vi "Vision Processor_modified.vi"(5 "error in":errorcluster, 7 "Image In":T2) -> (0 "error out":errorcluster, 3 "Image Out":T2(plugin-control))   [LabVIEW 2013]
uses:
  <vilib>/vision/Image Controls.llb/IMAQ Image.ctl
  <vilib>/vision/NI_Vision_Development_Module.lvlib
panel:
  out "HSL Histogram":T1(graph)
  out "Image In":T2(plugin-control)
  # "0  center of mass x\n1  center of mass y\n2  first pixel x\n3  first pixel y\n4  bounding rect left\n5  bounding rect top\n6  bounding rect right\n7  bounding rect bottom\n8 max feret diameter start x\n9  max feret diameter start y\n10 max feret diameter end x\n11 max feret diameter end y\n12 max horiz segment length left\n13 max horiz segment length right\n14 max horiz segment length row\n15 bounding rect width \n16 bounding rect height\n17 bounding rect diagional\n..\n33 area"
  # "13'3\"\n3'9\""
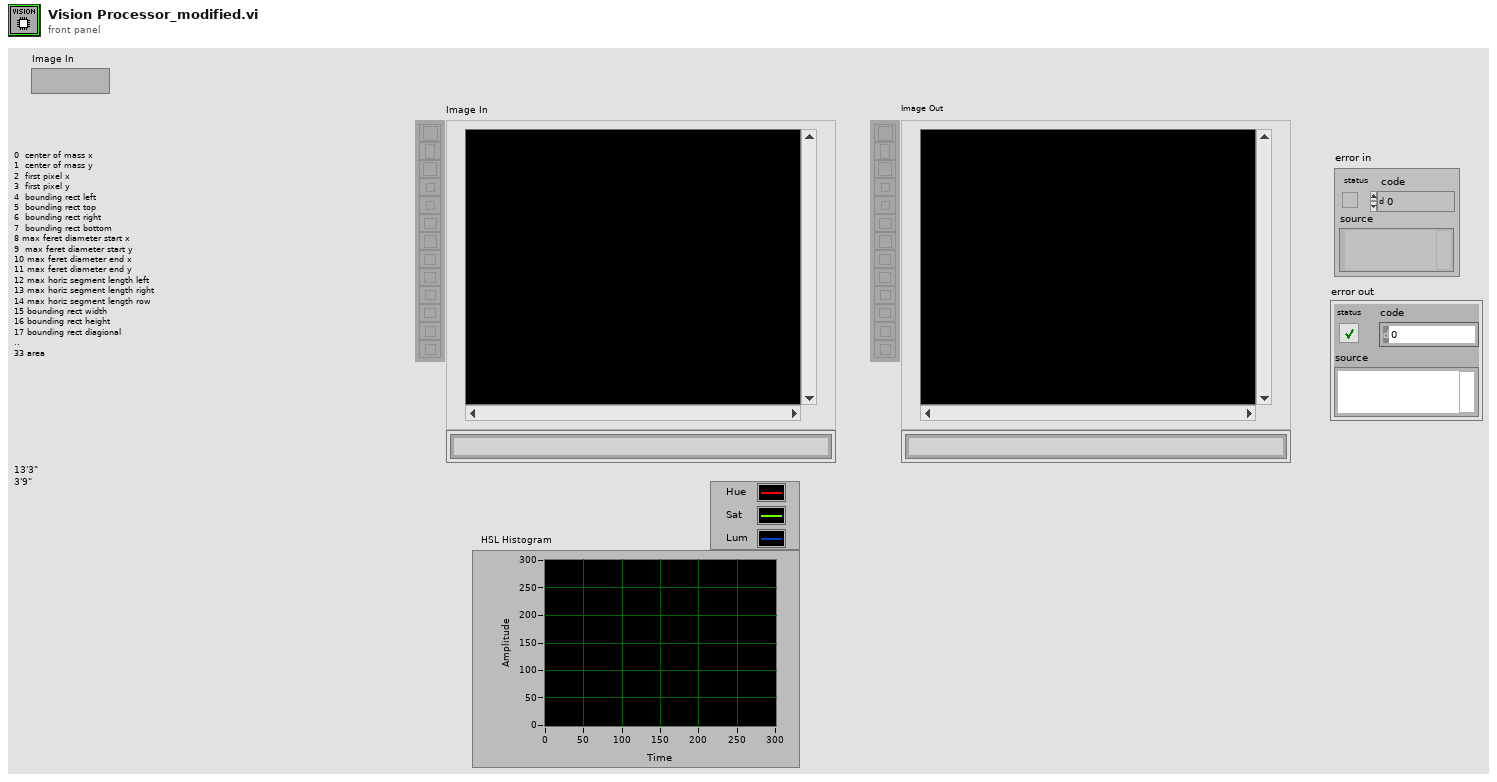
[diagram p1: front panel]
types:
  T1 = cluster{"Starting Value":sgl, "Incremental Value":sgl, "Histogram":u32[]}[]
  T2 = typedef "IMAQ Image.ctl" = refnum<image>
  T3 = enum32{"AutoM", "Close", "Dilate", "Erode", "Gradient", "Gradient out", "Gradient in", "Hit miss", "Open", "PClose", "POpen", "Thick", "Thin"}
  T4 = typedef "Image Type" = u32
  T5 = cluster{"Starting Value":sgl, "Incremental Value":sgl, "Histogram":u32[]}
  T6 = typedef "Particle Parameters" = i32
  T7 = cluster{"Measurement Parameter":T6, "Range Lower Value":dbl, "Range Upper Value":dbl, "Range":bool, "Measurement Type":bool}[]
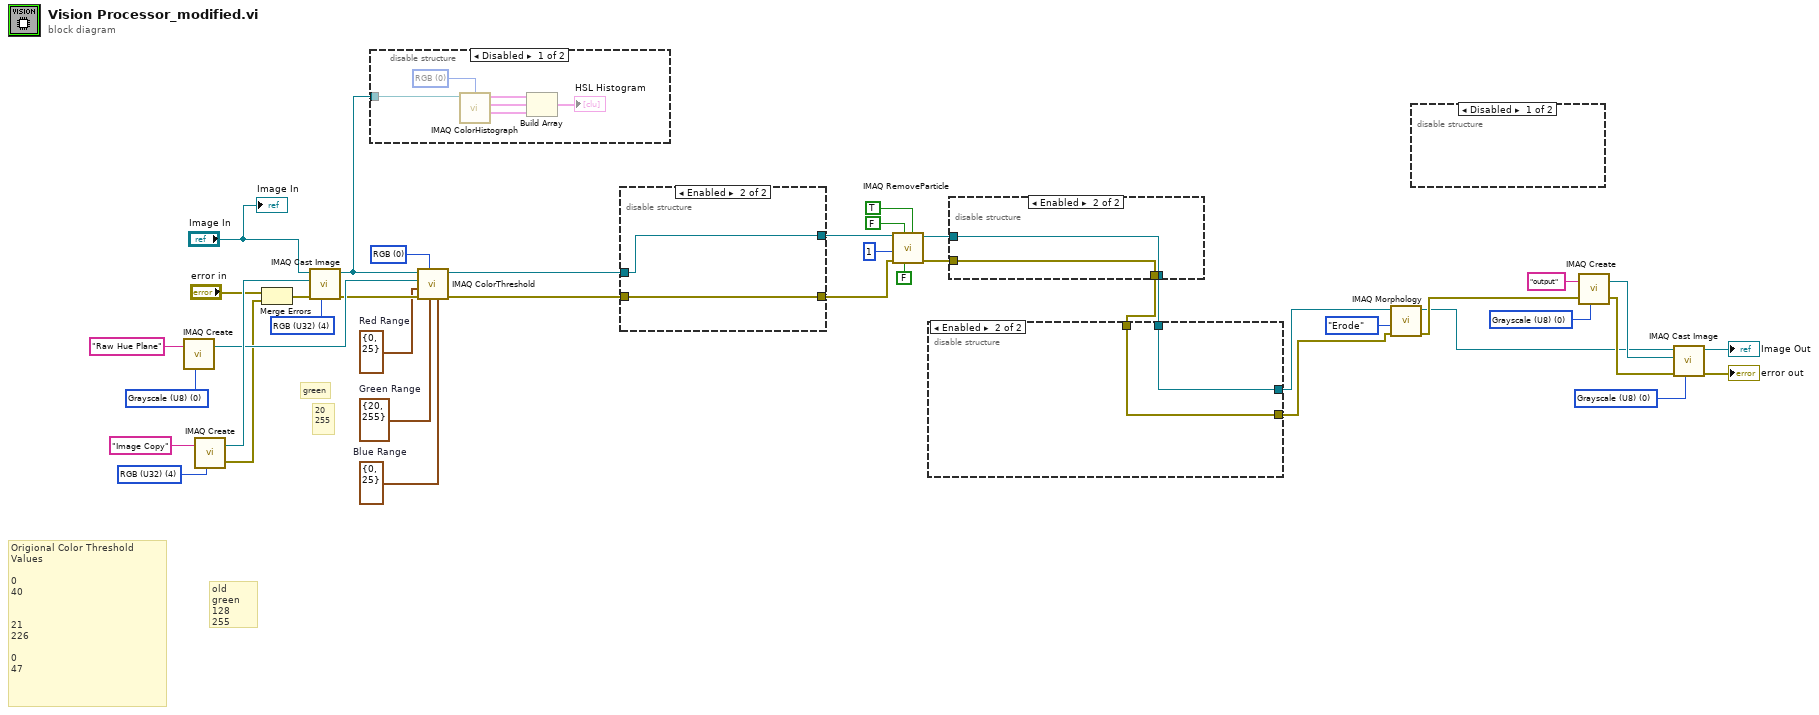
[diagram p0: block diagram]
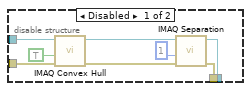
[diagram p2: hidden frame]
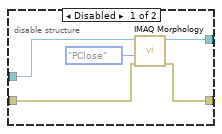
[diagram p3: hidden frame]
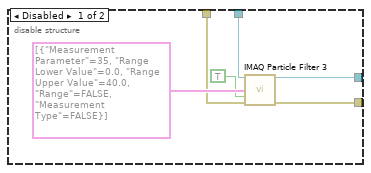
[diagram p5: hidden frame]
diagram:
  w12 = T4 0 items=["Grayscale (U8)", "Grayscale (I16)", "Grayscale (SGL)", "Complex (CSG)", "RGB (U32)", "HSL (U32)", "RGB (U64)", "Grayscale (U16)"] ("Image Type")
  w24 = T4 0 items=["Grayscale (U8)", "Grayscale (I16)", "Grayscale (SGL)", "Complex (CSG)", "RGB (U32)", "HSL (U32)", "RGB (U64)", "Grayscale (U16)"] ("Image Type")
  w25 = cluster{"Lower value":i32, "Upper value":i32} {"Lower value"=0, "Upper value"=25}  # Blue Range
  w28 = cluster{"Lower value":i32, "Upper value":i32} {"Lower value"=0, "Upper value"=25}  # Red Range
  w31 = cluster{"Lower value":i32, "Upper value":i32} {"Lower value"=20, "Upper value"=255}  # Green Range
  w29 = u16 0 items=["RGB", "HSL", "HSV", "HSI"] ("Color Mode")
  w37 = T4 0 items=["Grayscale (U8)", "Grayscale (I16)", "Grayscale (SGL)", "Complex (CSG)", "RGB (U32)", "HSL (U32)", "RGB (U64)", "Grayscale (U16)"] ("Image Type")
  w39 = T4 4 items=["Grayscale (U8)", "Grayscale (I16)", "Grayscale (SGL)", "Complex (CSG)", "RGB (U32)", "HSL (U32)", "RGB (U64)", "Grayscale (U16)"] ("Image Type")
  w40 = T4 4 items=["Grayscale (U8)", "Grayscale (I16)", "Grayscale (SGL)", "Complex (CSG)", "RGB (U32)", "HSL (U32)", "RGB (U64)", "Grayscale (U16)"] ("Image Type")
  # "old green\n128\n255"
  # "green"
  # "20\n255"
  # "Origional Color Threshold Values\n\n0\n40\n\n\n21\n226\n\n0\n47"
  n1 = call "IMAQ Create"("Image Name"="Raw Hue Plane", "Image Type"=w37) -> ("New Image"=w33:T2)  [unwired: 3 in, 1 out]
  n2 = call "IMAQ Create"("Image Name"="Image Copy", "Image Type"=w40) -> ("New Image"=w36:T2, "error out"=w26:errorcluster)  [unwired: 3 in]
  n3 = Merge Errors("error in", w26) -> (w27:errorcluster)
  n4 = call "IMAQ Cast Image"("Image Type"=w39, "error in (no error)"=w27, "Image Dst"=w36, "Image Src"="Image In") -> ("error out"=w30:errorcluster, "Image Dst Out"=w32:T2)  [unwired: 6 in]
  n5 = disable-structure shown="Disabled" {
    disable-tunnel: w32 -> [w42 _]
    frame Disabled {
      w43 = u16 0 items=["RGB", "HSL", "HSV", "HSI"] ("Color Mode")
      n6 = call "IMAQ ColorHistograph"("Color Mode"=w43, "Image Src"=w42) -> ("Red or Hue Histogram Graph"=w47:T5, "Green or Sat Histogram Graph"=w46:T5, "Blue or Luma or Val or Inten Histogram Graph"=w45:T5)  [unwired: 4 in, 1 out]
      n7 = Build Array(w47, w46, w45) -> (→"HSL Histogram":T1)
    }
    frame Enabled {
    }
  }
  n8 = call "IMAQ ColorThreshold"("Blue or Luma or Val or Inten Range"=w25, "Green or Sat Range"=w31, "Color Mode"=w29, "error in (no error)"=w30, "Red or Hue Range"=w28, "Image Dst"=w33, "Image Src"=w32) -> ("error out"=w16:errorcluster, "Image Dst Out"=w17:T2)  [unwired: 3 in]
  n9 = disable-structure shown="Enabled" {
    disable-tunnel: [w51 w54] -> w18
    disable-tunnel: w17 -> [w50 w54]
    disable-tunnel: w16 -> [w49 w53]
    disable-tunnel: [w48 w53] -> w15
    frame Disabled {
      n10 = call "IMAQ Morphology"("error in (no error)"=w49, "Operation"=T3."PClose", "Image Src"=w50) -> ("error out"=w48:errorcluster, "Image Dst Out"=w51:T2)  [unwired: 7 in]
    }
    frame Enabled {
    }
  }
  n11 = call "IMAQ RemoveParticle"("Connectivity 4/8 (8)"=TRUE, "Low Pass/High Pass (Low)"=FALSE, "Square/Hexa (Square)"=FALSE, "error in (no error)"=w15, "Number of Erosion"=1, "Image Src"=w18) -> ("error out"=w8:errorcluster, "Image Dst Out"=w9:T2)  [unwired: 1 in, 3 out]
  n12 = disable-structure shown="Enabled" {
    disable-tunnel: w9 -> [w61 w64]
    disable-tunnel: w8 -> [w60 w63]
    disable-tunnel: [w58 w64] -> w7
    disable-tunnel: [w55 w63] -> w6
    frame Disabled {
      n13 = call "IMAQ Convex Hull"("error in (no error)"=w60, "Connectivity 4/8 (8)"=TRUE, "Image Src"=w61) -> ("error out"=w56:errorcluster, "Image Dst Out"=w59:T2)  [unwired: 1 in, 6 out]
      n14 = call "IMAQ Separation"("error in (no error)"=w56, "Nb of Erosion"=1, "Image Src"=w59) -> ("error out"=w55:errorcluster, "Image Dst Out"=w58:T2)  [unwired: 7 in]
    }
    frame Enabled {
    }
  }
  n15 = disable-structure shown="Enabled" {
    disable-tunnel: w7 -> [w69 w72]
    disable-tunnel: [w67 w72] -> w3
    disable-tunnel: w6 -> [w66 w71]
    disable-tunnel: [w65 w71] -> w4
    frame Disabled {
      n16 = call "IMAQ Particle Filter 3"("Image Src"=w69, "Selection Values"=T7 [{"Measurement Parameter"=35, "Range Lower Value"=0.0, "Range Upper Value"=40.0, "Range"=FALSE, "Measurement Type"=FALSE}], "Keep/Remove Particles (F)"=TRUE, "error in (no error)"=w66) -> ("Image Dst Out"=w67:T2, "error out"=w65:errorcluster)  [unwired: 9 in, 1 out]
    }
    frame Enabled {
    }
  }
  n17 = call "IMAQ Morphology"("error in (no error)"=w4, "Operation"=T3."Erode", "Image Src"=w3) -> ("error out"=w2:errorcluster, "Image Dst Out"=w1:T2)  [unwired: 7 in]
  n18 = disable-structure shown="Disabled" {
    frame Disabled {
    }
    frame Enabled {
    }
  }
  n19 = call "IMAQ Create"("Image Name"="output", "Image Type"=w24, "error in (no error)"=w2) -> ("New Image"=w14:T2, "error out"=w13:errorcluster)  [unwired: 2 in]
  n20 = call "IMAQ Cast Image"("Image Type"=w12, "error in (no error)"=w13, "Image Dst"=w14, "Image Src"=w1) -> ("error out"=→"error out":errorcluster, "Image Dst Out"=→"Image Out":T2)  [unwired: 6 in]
  "Image In" <- "Image In"
